vi "File Washer HCC.vi"(0 "Washer Array":T1[](array[typedef]), 1 "Dryer s,h Data Dir":path, 2 "Header":string[][](array[string]), 5 "Dryer Bank Filename":path, 7 "Data Set ID":string="Test Station A-G", 9 "Last Save Hour":string="Aisle1", 11 "error in (no error)":errorcluster, 12 "Sample Data Current Filename":path) -> (4 "Dryer Aisle Out":T3[](array[typedef]) {"Cycle Count" format="%05d"}, 6 "Last Save Hour Out":string, 8 "Sample Data Current Filename Out":path, 15 "error out":errorcluster)   [LabVIEW 2011]
uses:
  Washer.ctl
  Dryer Wilt/Dryer Details.ctl
  HCC Data.ctl
  Washer Status Ctrl.ctl
panel:
  in  "Stop":bool=TRUE
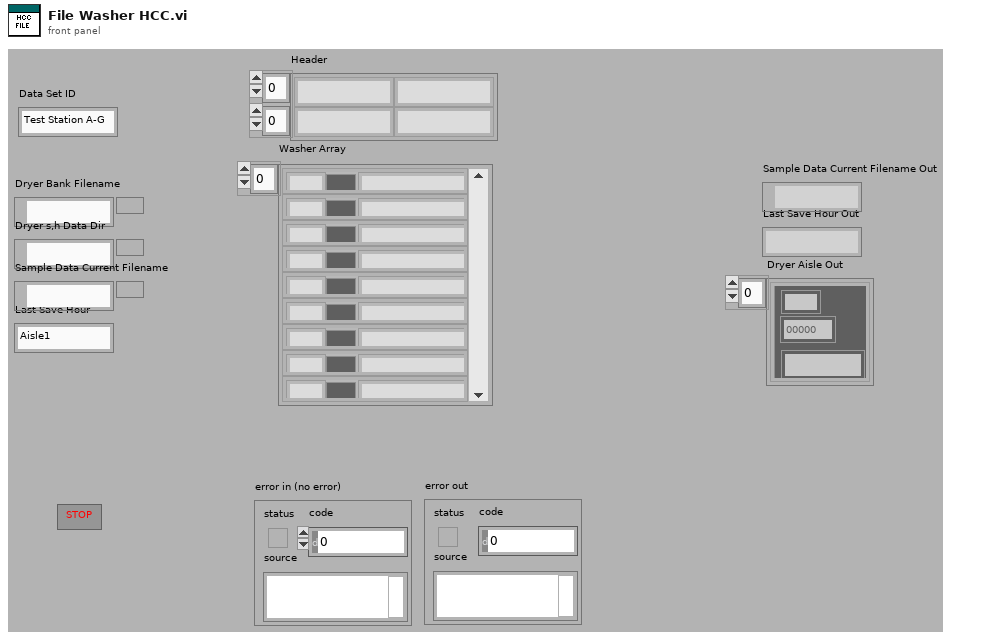
[diagram p1: front panel]
types:
  T1 = typedef "HCC Data.ctl" = cluster{"Station":string, "Color":u32, "Status":T2, "Error Time":string, "Com Err Count":u32, "Debug Log":string}
  T2 = typedef "Washer Status Ctrl.ctl" = enum16{"Running", "Err", "No Com", "No Conf"}
  T3 = typedef "Washer.ctl" = cluster{"Serial Number":string, "Cycle Count":i32, "Station Number":string, "Dryer Details":T4, "Sample Record(t, CC, ASCII, Status ) ":string[], "Hist Record(Cycle Count, t-comp) ":string[][], "Status Color":u32, "Com Port":u8, "Bad Com Count":i32, "Boolean":bool}
  T4 = typedef "Dryer Details.ctl" = cluster{"Station":string, "Cycle Count Day":string, "Status":string, "Debug ASCII":string, "Notes":string, "Serial Number":string, "Total Time On":string, "TR Number":string, "Cycle Count Night":string, "Time On Day":string, "Time On Night":string}
  T5 = enum32{"Invalid", "Standard", "Closed", "Hidden", "Minimized", "Maximized"}
  T6 = enum16{"Read 2D Array", "Write 2D Array", "Write/Append 1D Array"}
  T7 = cluster{"This VI":refnum<vi>, "Washer Array":T1[], "Dryer Bank Filename":path, "Dryer Aisle Ot":T3[], "Dryer s,h Data Dir":path, "Last Save Hour":string, "Sample Data Current Filename":path, "All Sample Data":string[][], "Data Set ID":string}
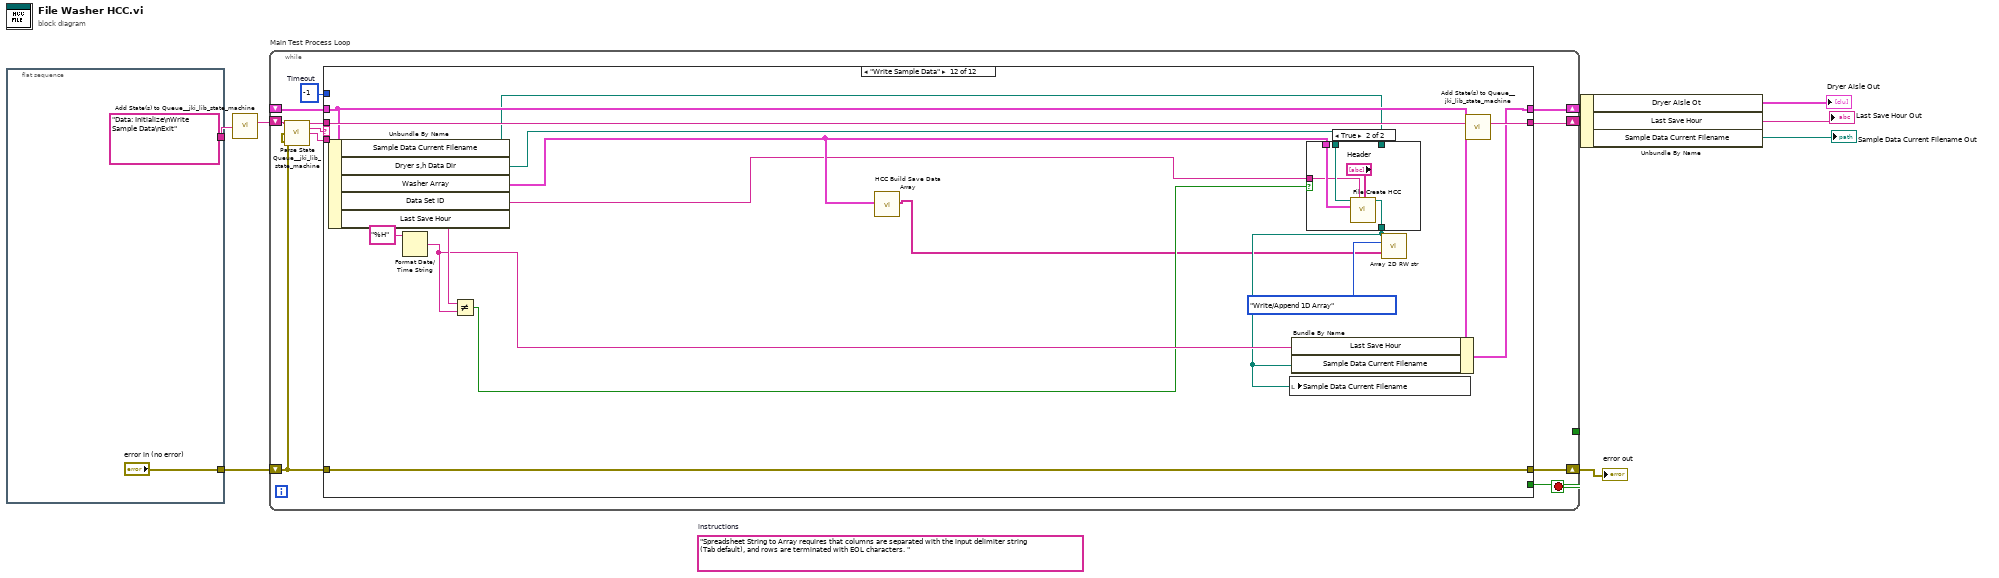
[diagram p0: block diagram]
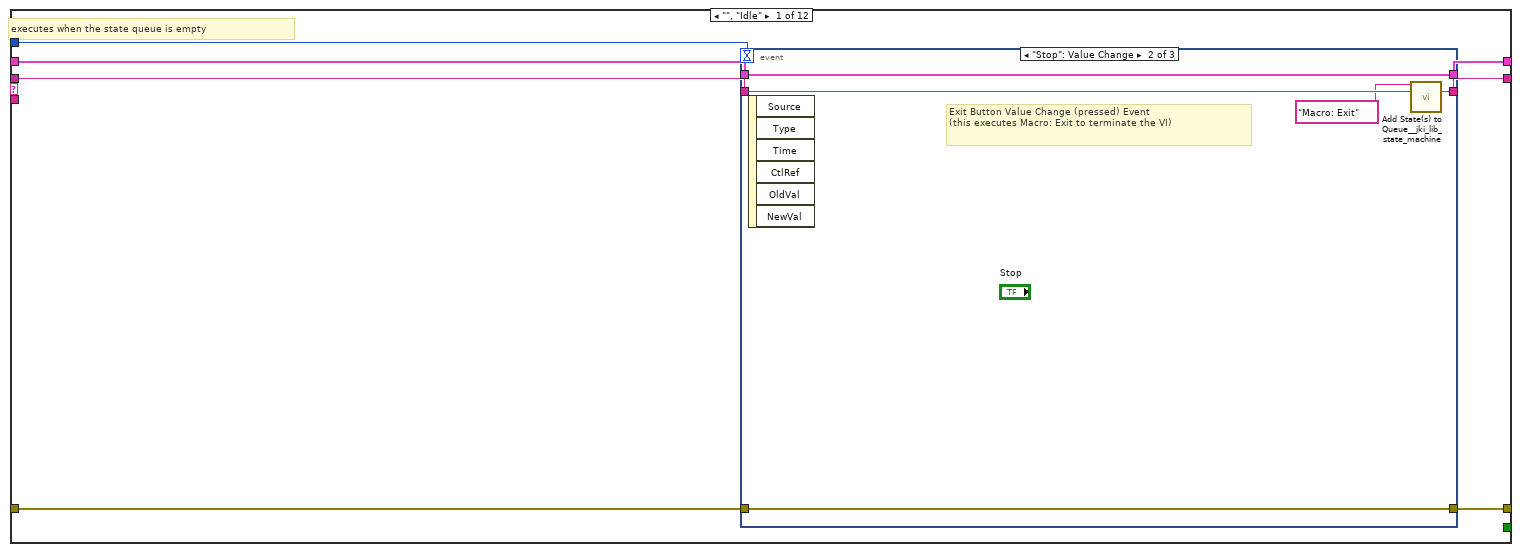
[diagram p2: hidden frame]
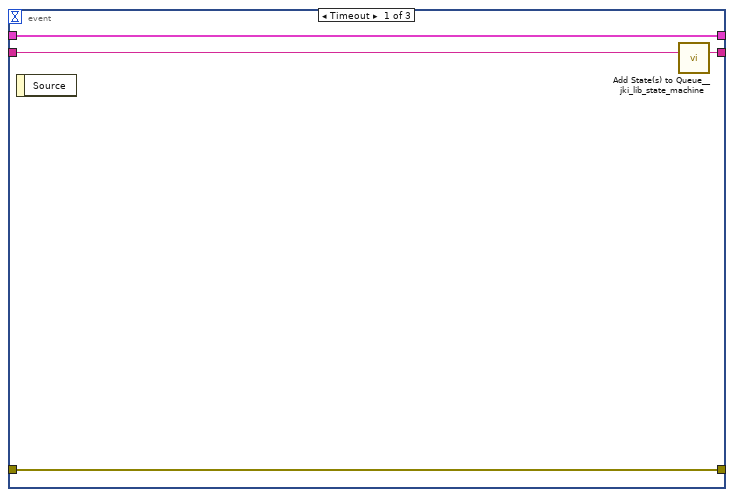
[diagram p3: hidden frame]
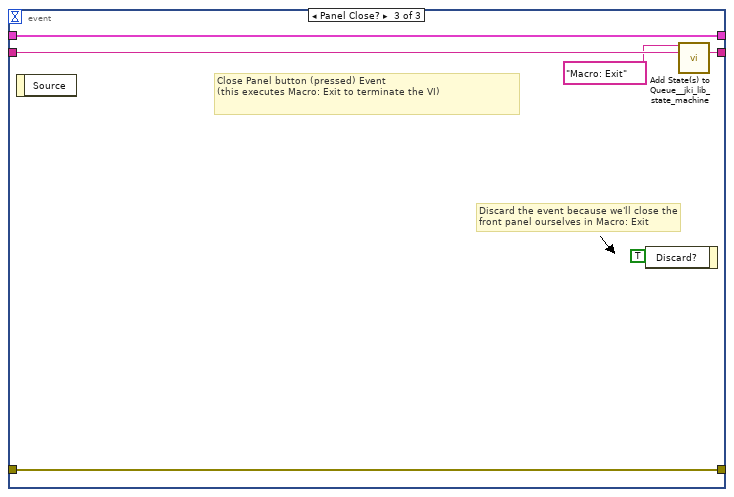
[diagram p4: hidden frame]
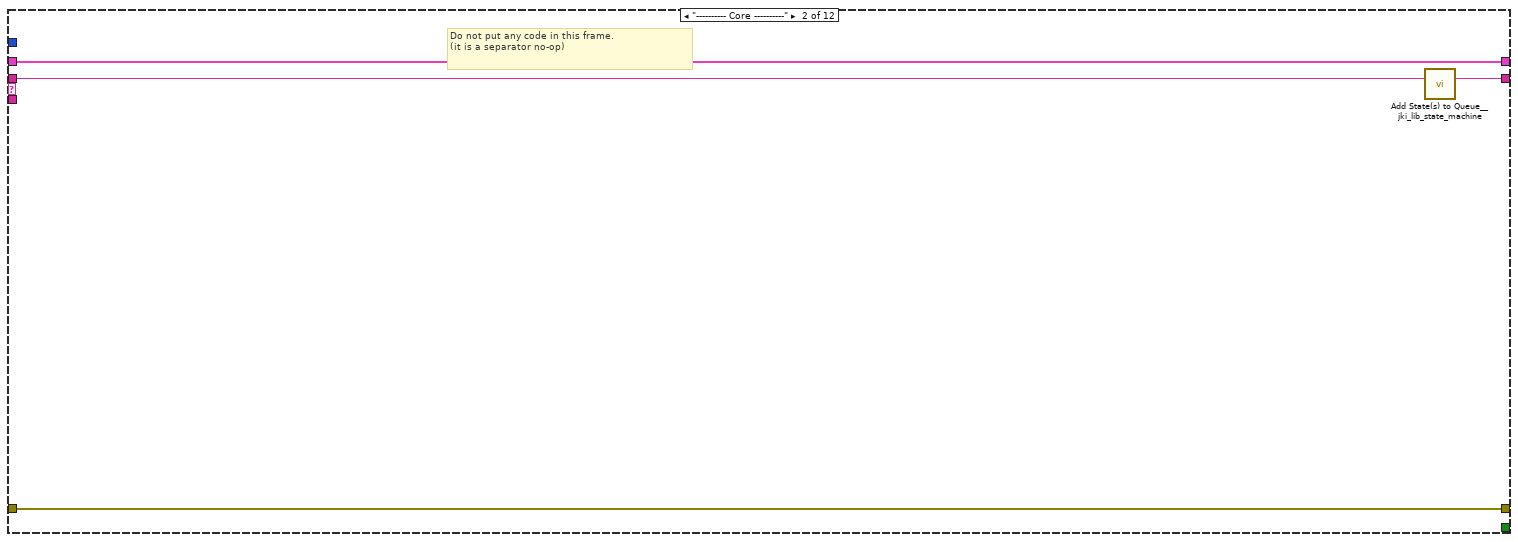
[diagram p5: hidden frame]
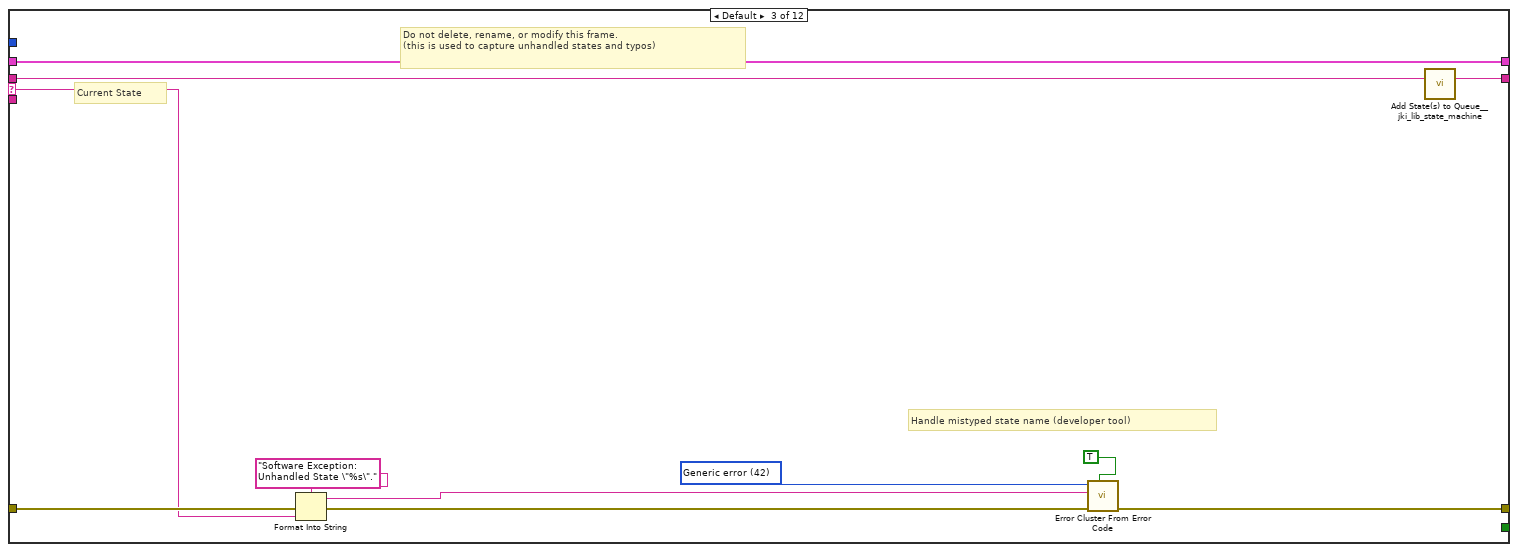
[diagram p6: hidden frame]
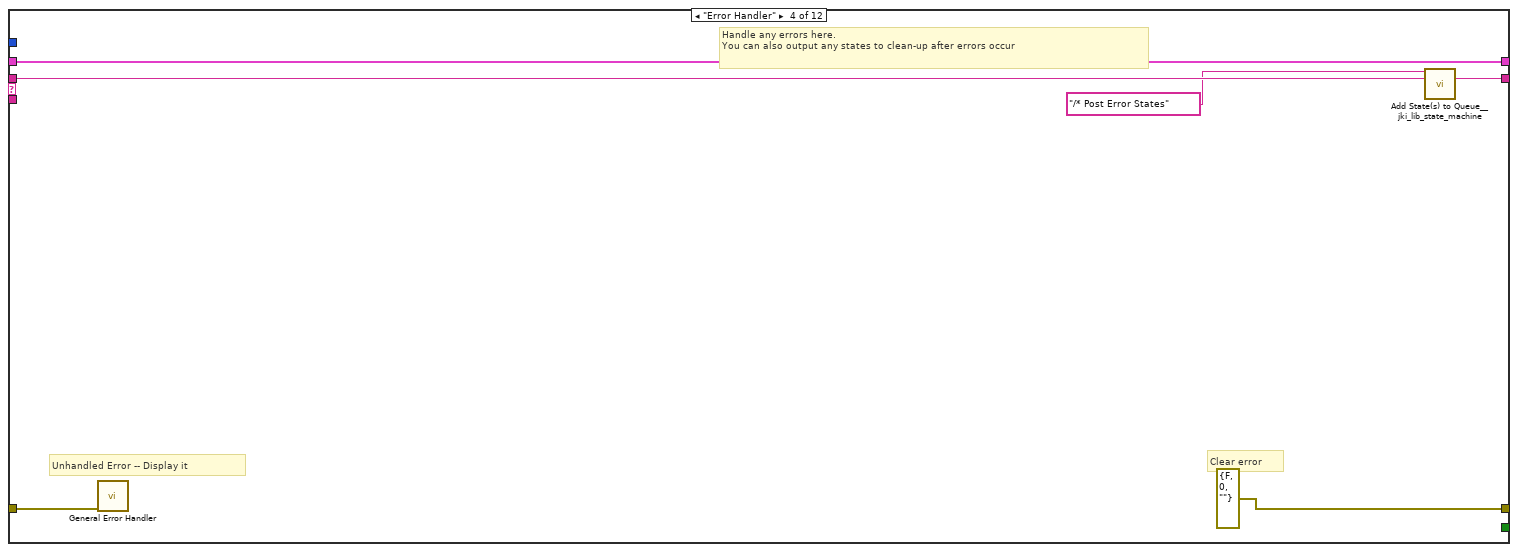
[diagram p7: hidden frame]
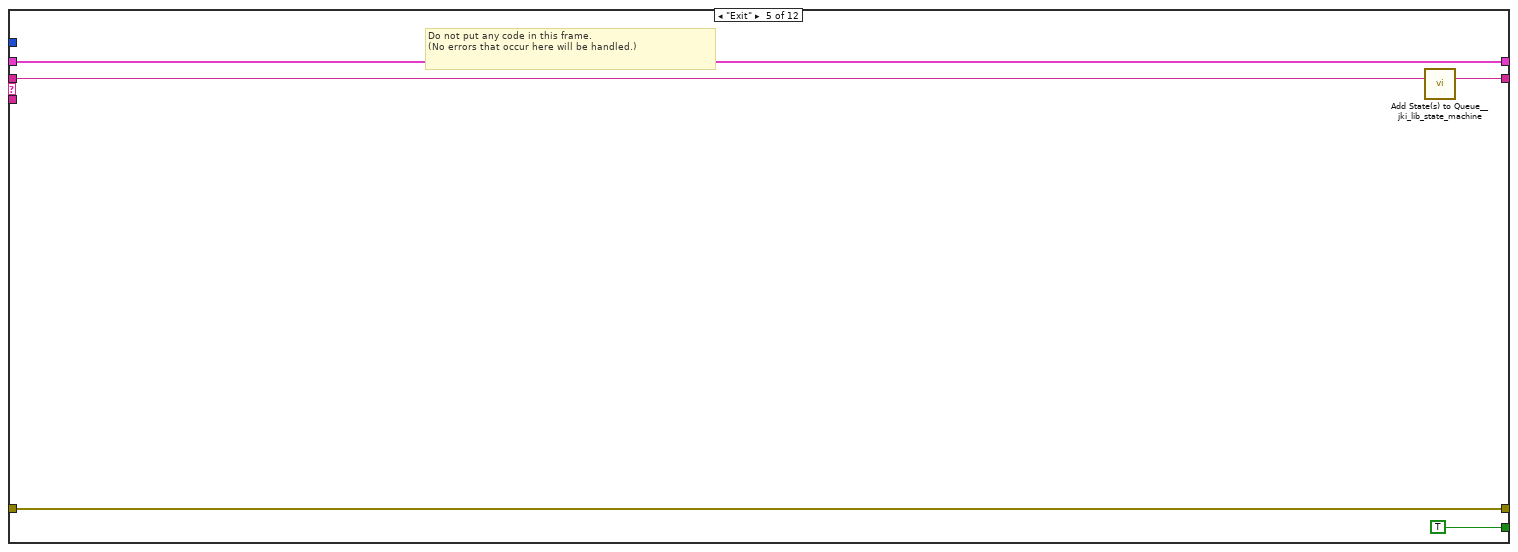
[diagram p8: hidden frame]
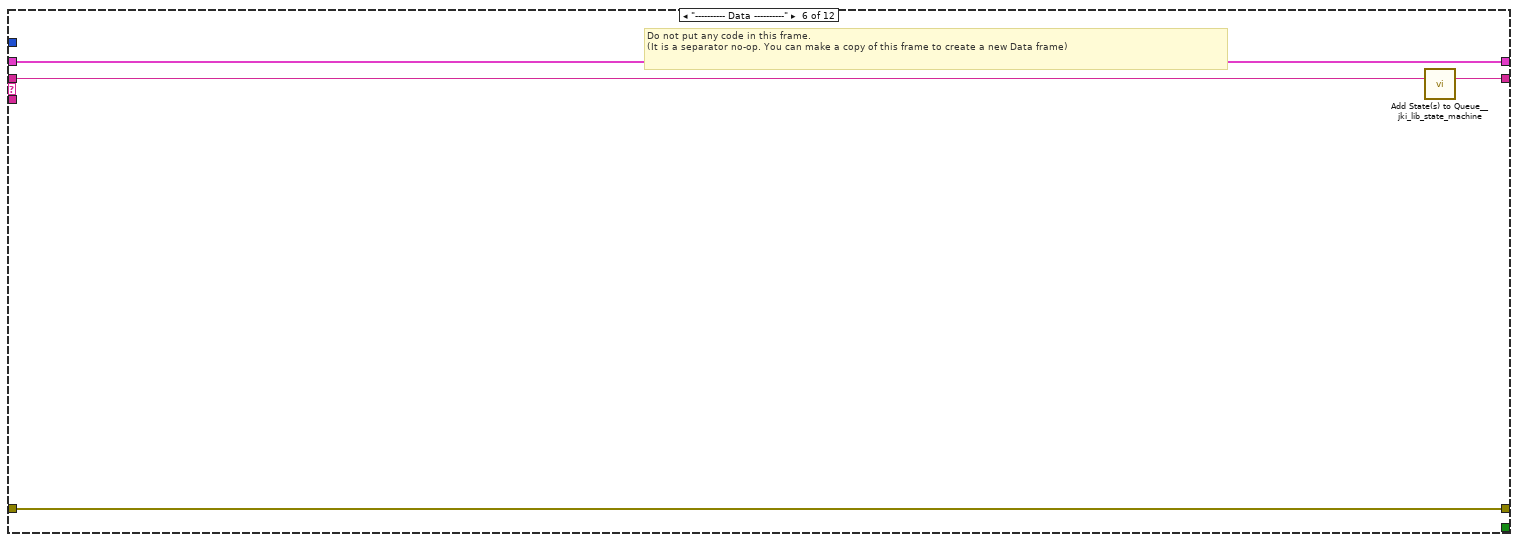
[diagram p9: hidden frame]
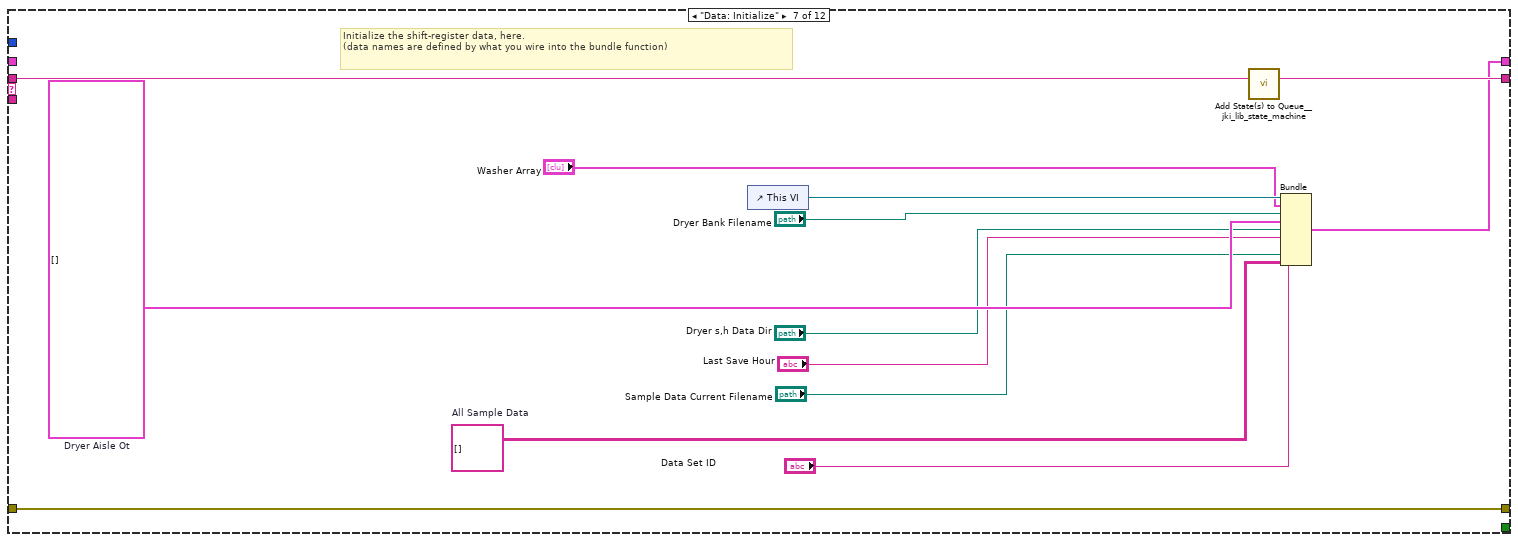
[diagram p10: hidden frame]
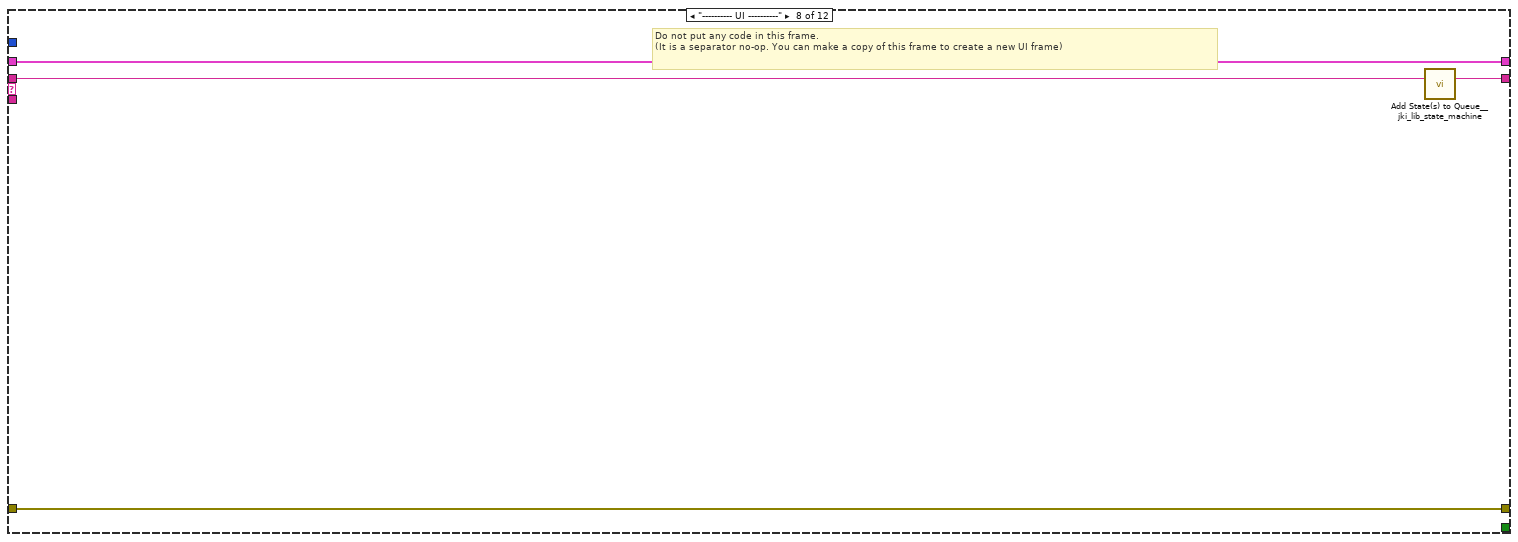
[diagram p11: hidden frame]
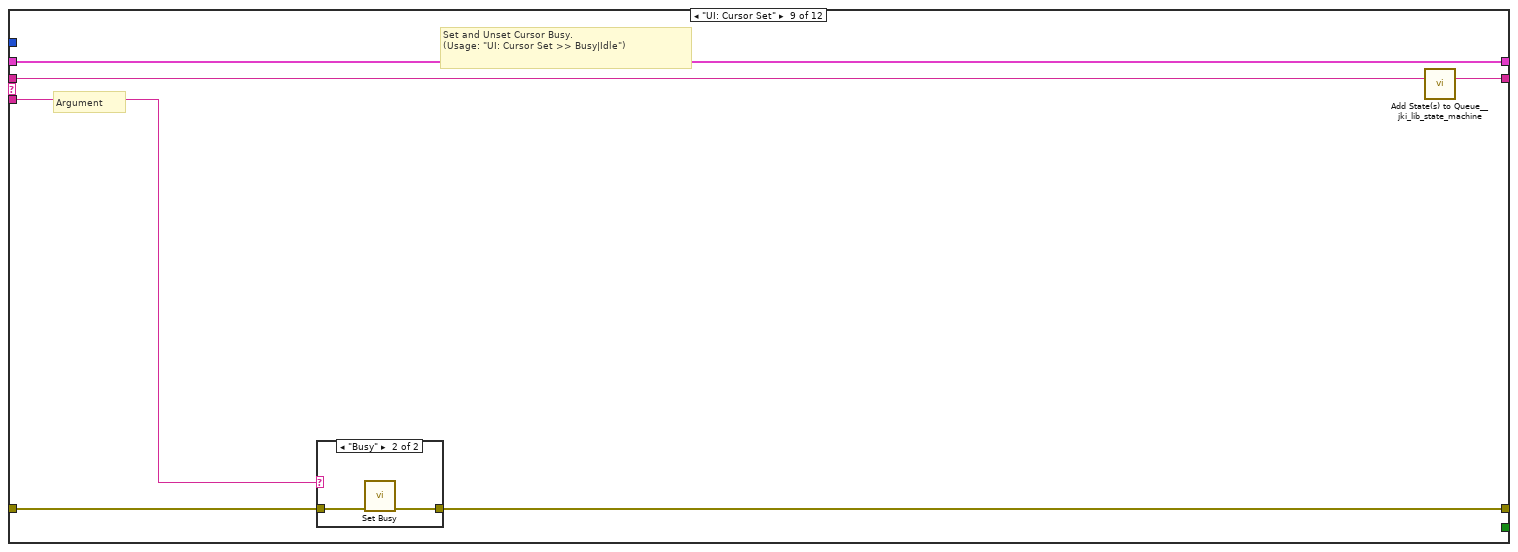
[diagram p12: hidden frame]
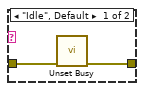
[diagram p13: hidden frame]
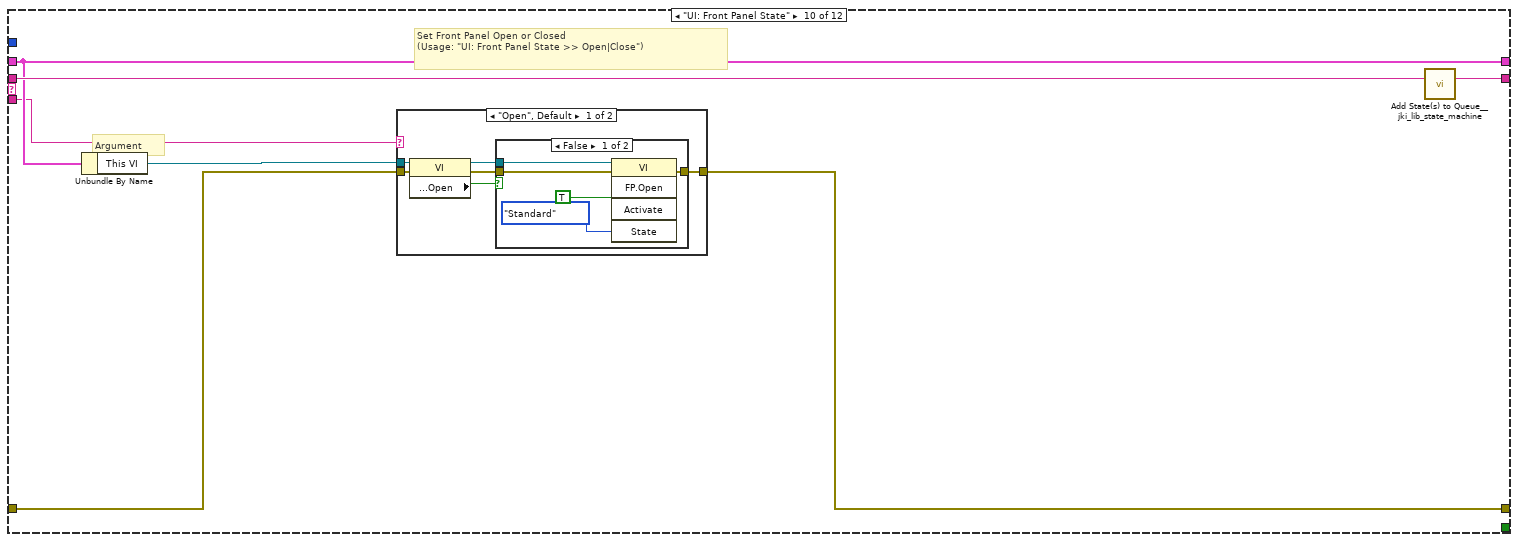
[diagram p14: hidden frame]
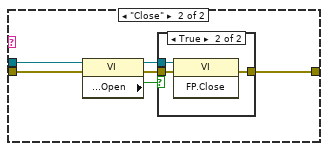
[diagram p16: hidden frame]
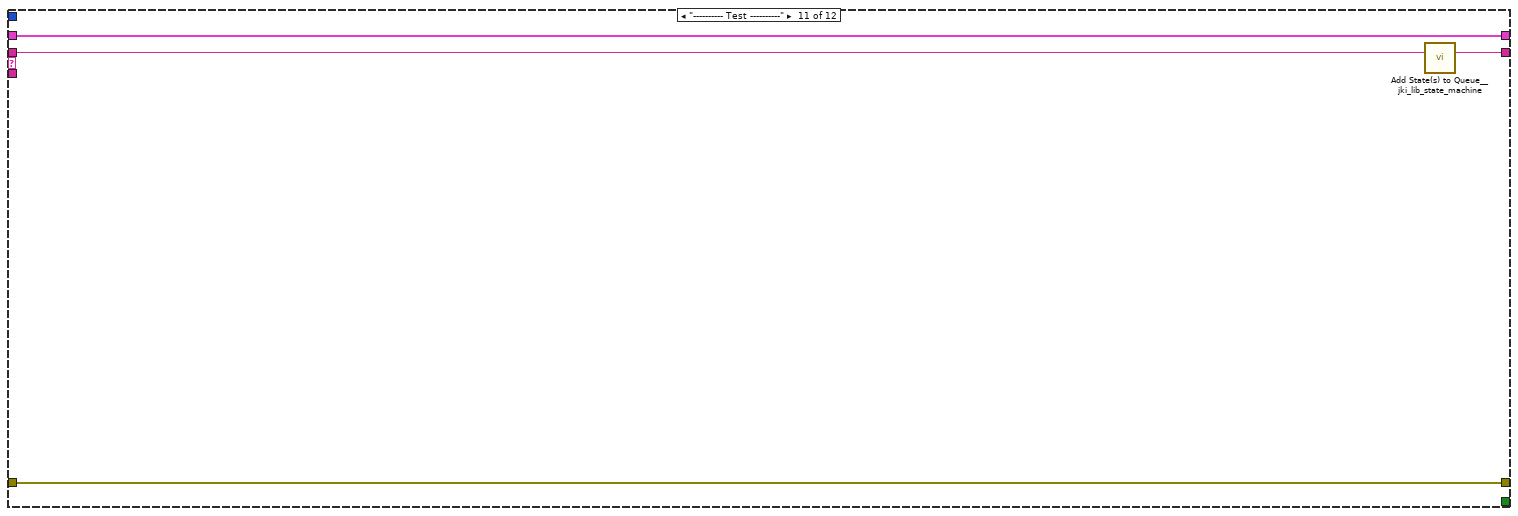
[diagram p18: hidden frame]
diagram:
  (unwired) "Spreadsheet String to Array requires that columns are separated with the input delimiter string (Tab default), and rows are terminated with EOL characters. "  # instructions
  n1 = flat-sequence {
    tunnel: ["Data: Initialize\nWrite Sample Data\nExit"] -> w7
    tunnel: ["error in (no error)"] -> w3
    frame #0 {
    }
  }
  n2 = call <vilib>:"Add State(s) to Queue__jki_lib_state_machine.vi"("State(s) at Back (\"\")"=w7) -> ("States Out"=w8:string)  [unwired: 14 in]
  n3 = while "Main Test Process Loop" {
    shift-right: [w15] -> w6
    shift-left: _ -> [w14]
    shift-right: [w17] -> w4
    shift-left: w3 -> [w12]
    shift-right: [w16] -> _
    shift-left: w8 -> [w18]
    tunnel: [w11] -> _
    stop <- w11 stop-if-true
    w13 = -1  # Timeout
    n4 = call <vilib>:"Parse State Queue__jki_lib_state_machine.vi"("State Queue"=w18, "Error In (no error)"=w12) -> ("Remaining States"=w20:string, "Current State"=w21:string, "Arguments"=w19:string)  [unwired: 11 in]
    n5 = case shown="\"Write Sample Data\"" w21 {
      selector: w21 -> [_ _ w48 _ _ _ _ _ _ _ _ _]
      tunnel: w20 -> [w28 w47 w52 w64 w69 w73 w86 w90 w96 w107 w133 w149]
      tunnel: w19 -> [_ _ _ _ _ _ _ _ w91 w101 _ _]
      tunnel: w14 -> [w26 w44 w50 w61 w67 w70 _ w87 w94 w103 w130 w143]
      tunnel: [w25 w45 w54 errorcluster {"status"=FALSE, "code"=0, "source"=""} ("error out") w66 w71 w83 w88 w92 w104 w131 w147] -> w17
      tunnel: w12 -> [w24 w45 w53 w60 w66 w71 w83 w88 w93 w105 w131 w147]
      tunnel: [w27 w46 w51 w63 w68 w72 w85 w89 w95 w106 w132 w148] -> w16
      tunnel: [_ _ _ _ TRUE _ _ _ _ _ _ _] -> w11
      tunnel: [w23 w44 w50 w61 w67 w70 w84 w87 w94 w103 w130 w142] -> w15
      tunnel: w13 -> [w22 _ _ _ _ _ _ _ _ _ _ _]
      frame "", "Idle" {
        # "executes when the state queue is empty"
        n6 = event shown="[1] \"Stop\": Value Change" {
          selector: _ -> [_ _ _]
          dyn-events: _ -> [_ _ _]
          timeout: w22 -> [_ _ _]
          tunnel: w28 -> [w32 w37 w43]
          tunnel: [w31 w36 w42] -> w27
          tunnel: w26 -> [w29 w34 w40]
          tunnel: [w30 w35 w41] -> w25
          tunnel: w24 -> [w30 w35 w41]
          tunnel: [w29 w34 w40] -> w23
          event Timeout {
            n7 = event-data() -> ()  [unwired: 1 in, 1 out]
            n8 = call <vilib>:"Add State(s) to Queue__jki_lib_state_machine.vi"("State(s) in (\"\")"=w32) -> ("States Out"=w31:string)  [unwired: 14 in]
          }
          event "Stop": Value Change {
            # "Exit Button Value Change (pressed) Event\n(this executes Macro: Exit to terminate the VI)"
            n9 = event-data() -> ()  [unwired: 1 in, 6 out]
            n10 = call <vilib>:"Add State(s) to Queue__jki_lib_state_machine.vi"("State(s) in Front (\"\")"="Macro: Exit", "State(s) in (\"\")"=w37) -> ("States Out"=w36:string)  [unwired: 13 in]
          }
          event Panel Close? {
            # "Discard the event because we'll close the front panel ourselves in Macro: Exit"
            # "Close Panel button (pressed) Event\n(this executes Macro: Exit to terminate the VI)"
            n11 = event-data() -> ()  [unwired: 1 in, 1 out]
            n12 = event-data("Discard?"=TRUE) -> ()  [unwired: 1 in, 1 out]
            n13 = call <vilib>:"Add State(s) to Queue__jki_lib_state_machine.vi"("State(s) in Front (\"\")"="Macro: Exit", "State(s) in (\"\")"=w43) -> ("States Out"=w42:string)  [unwired: 13 in]
          }
        }
      }
      frame "---------- Core ----------" {
        # "Do not put any code in this frame.\n(it is a separator no-op)"
        n14 = call <vilib>:"Add State(s) to Queue__jki_lib_state_machine.vi"("State(s) in (\"\")"=w47) -> ("States Out"=w46:string)  [unwired: 14 in]
      }
      frame Default {
        w57 = 42 items=["No error", "Argument error", "Memory is full", "Out of zone", "End of file", "File already open", "Generic file I/O error", "File not found", "File permission error", "Disk is full", "Duplicate path", "Too many files open", "System feature not enabled", "Resource file not found", "Cannot add resource", "Resource not found", "Image not found", "Image memory error", "Pen does not exist", "Config type invalid", "Config token not found", "Config parse error", "Config memory error", "Bad external code format", "Bad external code offset", "External code not present", "Null window", "Destroy window error", "Null menu", "Print aborted", "Bad print record", "Print driver error", "Windows error during printing", "Memory error during printing", "Print dialog error", "Generic print error", "Invalid device refnum", "Device not found", "Device parameter error", "Device unit error", "Cannot open device", "Device call aborted", "Generic error", "Cancelled by user", "Object ID too low", "Object ID too high", "Object not in heap", "Unknown heap", "Unknown object (invalid DefProc)", "Unknown object (DefProc not in table)", "Message out of range", "Invalid (null) method", "Unknown message", "Manager call not supported", "Bad address", "Network operation in progress", "Network operation timed out", "Connection is busy", "Network attribute not supported", "Network error", "Address in use", "System out of memory", "Connection aborted", "Connection refused", "Not connected", "Already connected", "Connection closed", "Initialization error (interapplication manager)", "Bad occurrence", "Wait on unbound occurrence handler", "Occurrence queue overflow", "Datalog type conflict", "Unused", "Unrecognized type (interapplication manager)", "Memory corrupt", "Failed to make temporary DLL", "Old CIN version", "Drag socket not found", "Failed to load drop-object", "Failed to register OLE object", "Failed to release OLE object", "Format specifier type mismatch", "Unknown format specifier", "Too few format specifiers", "Too many format specifiers", "Scan failed", "Newer CIN version", "Error converting to variant", "Runtime menu error", "Password tampered", "Variant attribute not found", "Incompatible variant data type", "Event data is not available", "Event Store is not present", "Occurrence is not found", "Event Queue is not created", "Event info is not available", "Refnum passed is NULL", "Error retrieving Class GUID", "Error retrieving CoClass GUID", "Error retrieving TypeLib GUID.", "Bad built application magic bytes.", "Specific driver is different from the specific driver associated with the Logical Name.", "There is no session opened to the class driver.", "Max Error", "MAX - Error with config objects", "MAX - Error loading configuration", "MAX - Group not supported"]
        # "Current State"
        # "Do not delete, rename, or modify this frame.\n(this is used to capture unhandled states and typos)"
        # "Handle mistyped state name (developer tool)"
        n15 = Format Into String(format string="Software Exception: Unhandled State \"%s\"." ("message"), error in=w53, w48) -> (resulting string=w56:string, error out=w55:errorcluster)  [unwired: 1 in]
        n16 = call <vilib>:"Error Cluster From Error Code.vi"("show call chain? (False)"=TRUE, "error in (no error)"=w55, "error message (\"\")"=w56, "error code (0)"=w57) -> ("error out"=w54:errorcluster)  [unwired: 5 in]
        n17 = call <vilib>:"Add State(s) to Queue__jki_lib_state_machine.vi"("State(s) in (\"\")"=w52) -> ("States Out"=w51:string)  [unwired: 14 in]
      }
      frame "Error Handler" {
        # "Unhandled Error -- Display it"
        # "Handle any errors here.\nYou can also output any states to clean-up after errors occur"
        # "Clear error"
        n18 = call <vilib>:"General Error Handler.vi"("error in (no error)"=w60) -> ()  [unwired: 10 in, 5 out]
        n19 = call <vilib>:"Add State(s) to Queue__jki_lib_state_machine.vi"("State(s) in Front (\"\")"="/* Post Error States", "State(s) in (\"\")"=w64) -> ("States Out"=w63:string)  [unwired: 13 in]
      }
      frame "Exit" {
        # "Do not put any code in this frame.\n(No errors that occur here will be handled.)"
        n20 = call <vilib>:"Add State(s) to Queue__jki_lib_state_machine.vi"("State(s) in (\"\")"=w69) -> ("States Out"=w68:string)  [unwired: 14 in]
      }
      frame "---------- Data ----------" {
        # "Do not put any code in this frame.\n(It is a separator no-op. You can make a copy of this frame to create a new Data frame)"
        n21 = call <vilib>:"Add State(s) to Queue__jki_lib_state_machine.vi"("State(s) in (\"\")"=w73) -> ("States Out"=w72:string)  [unwired: 14 in]
      }
      frame "Data: Initialize" {
        w76 = string[][] []  # All Sample Data
        w81 = T3[] []  # Dryer Aisle Ot
        # "Initialize the shift-register data, here.\n(data names are defined by what you wire into the bundle function)"
        n22 = control-ref of="This VI"() -> (w80:refnum<vi>)
        n23 = call <vilib>:"Add State(s) to Queue__jki_lib_state_machine.vi"("State(s) in (\"\")"=w86) -> ("States Out"=w85:string)  [unwired: 14 in]
        n24 = Bundle("This VI"=w80, "Washer Array"="Washer Array", "Dryer Bank Filename"="Dryer Bank Filename", "Dryer Aisle Ot"=w81, "Dryer s,h Data Dir"="Dryer s,h Data Dir", "Last Save Hour"="Last Save Hour", "Sample Data Current Filename"="Sample Data Current Filename", "All Sample Data"=w76, "Data Set ID"="Data Set ID") -> (w84:T7)  [unwired: 1 in]
      }
      frame "---------- UI ----------" {
        # "Do not put any code in this frame.\n(It is a separator no-op. You can make a copy of this frame to create a new UI frame)"
        n25 = call <vilib>:"Add State(s) to Queue__jki_lib_state_machine.vi"("State(s) in (\"\")"=w90) -> ("States Out"=w89:string)  [unwired: 14 in]
      }
      frame "UI: Cursor Set" {
        # "Argument"
        # "Set and Unset Cursor Busy.\n(Usage: \"UI: Cursor Set >> Busy|Idle\")"
        n26 = case shown="\"Busy\"" w91 {
          tunnel: w93 -> [w98 w100]
          tunnel: [w97 w99] -> w92
          frame "Idle", Default {
            n27 = call <vilib>:"Unset Busy.vi"("error in (no error)"=w98) -> ("error out"=w97:errorcluster)  [unwired: 10 in]
          }
          frame "Busy" {
            n28 = call <vilib>:"Set Busy.vi"("error in (no error)"=w100) -> ("error out"=w99:errorcluster)  [unwired: 9 in, 1 out]
          }
        }
        n29 = call <vilib>:"Add State(s) to Queue__jki_lib_state_machine.vi"("State(s) in (\"\")"=w96) -> ("States Out"=w95:string)  [unwired: 14 in]
      }
      frame "UI: Front Panel State" {
        # "Argument"
        # "Set Front Panel Open or Closed\n(Usage: \"UI: Front Panel State >> Open|Close\")"
        n30 = Unbundle By Name(w103) -> ("This VI"=w102:refnum<vi>)
        n31 = case shown="\"Open\", Default" w101 {
          tunnel: w105 -> [w111 w124]
          tunnel: [w113 w125] -> w104
          tunnel: w102 -> [w112 w122]
          frame "Open", Default {
            n32 = property class="VI"(reference=w112, error in=w111) -> (reference out=w109:refnum<vi>, error out=w110:errorcluster, "Front Panel.Open"=w108:bool)
            n33 = case shown="False" w108 {
              tunnel: [w116 w119] -> w113
              tunnel: w110 -> [w115 w119]
              tunnel: w109 -> [w114 _]
              frame False {
                n34 = invoke class="VI" method="FP.Open"(reference=w114, error in=w115, "Activate"=TRUE, "State"=T5."Standard") -> (error out=w116:errorcluster)  [unwired: 1 in, 4 out]
              }
              frame True {
              }
            }
          }
          frame "Close" {
            n35 = property class="VI"(reference=w122, error in=w124) -> (reference out=w121:refnum<vi>, error out=w123:errorcluster, "Front Panel.Open"=w120:bool)
            n36 = case shown="True" w120 {
              tunnel: [w126 w129] -> w125
              tunnel: w123 -> [w126 w128]
              tunnel: w121 -> [_ w127]
              frame False {
              }
              frame True {
                n37 = invoke class="VI" method="FP.Close"(reference=w127, error in=w128) -> (error out=w129:errorcluster)  [unwired: 1 in, 2 out]
              }
            }
          }
        }
        n38 = call <vilib>:"Add State(s) to Queue__jki_lib_state_machine.vi"("State(s) in (\"\")"=w107) -> ("States Out"=w106:string)  [unwired: 14 in]
      }
      frame "---------- Test ----------" {
        n39 = call <vilib>:"Add State(s) to Queue__jki_lib_state_machine.vi"("State(s) in (\"\")"=w133) -> ("States Out"=w132:string)  [unwired: 14 in]
      }
      frame "Write Sample Data" {
        n40 = Unbundle By Name(w143) -> ("Sample Data Current Filename"=w139:path, "Dryer s,h Data Dir"=w146:path, "Washer Array"=w136:T1[], "Data Set ID"=w134:string, "Last Save Hour"=w145:string)
        n41 = Format Date/Time String(time format string (%c)="%H") -> (date/time string=w141:string)  [unwired: 2 out]
        n42 = Not Equal?(x=w145, y=w141) -> (x != y?=w140:bool)
        n43 = call "HCC Build Save Data Array.vi"("Washer Array"=w136) -> ("appended array"=w135:string[])  [unwired: 10 in]
        n44 = case shown="True" w140 {
          tunnel: w136 -> [_ w153]
          tunnel: w146 -> [_ w155]
          tunnel: [w150 w154] -> w138
          tunnel: w139 -> [w150 _]
          tunnel: w134 -> [_ w152]
          frame False {
          }
          frame True {
            n45 = call "File Create HCC.vi"("base path"=w155, "Station,Data Set ID"=w152, "Header"="Header", "Washer Array"=w153) -> ("appended path"=w154:path)  [unwired: 11 in]
          }
        }
        n46 = local write "Sample Data Current Filename"(w138) -> ()
        n47 = Bundle By Name(cluster=w143, "Last Save Hour"=w141, "Sample Data Current Filename"=w138) -> (w142:T7)
        n48 = call "Array 2D RW str.vi"("file path (dialog if empty)"=w138, "Write/Read"=T6."Write/Append 1D Array", "1D Sample Append Array"=w135) -> ()  [unwired: 12 in, 1 out]
        n49 = call <vilib>:"Add State(s) to Queue__jki_lib_state_machine.vi"("State(s) in (\"\")"=w149) -> ("States Out"=w148:string)  [unwired: 14 in]
      }
    }
  }
  "error out" <- w4
  n50 = Unbundle By Name(w6) -> ("Dryer Aisle Ot"=→"Dryer Aisle Out":T3[], "Last Save Hour"=→"Last Save Hour Out":string, "Sample Data Current Filename"=→"Sample Data Current Filename Out":path)
